vi "Pump Elapsed Time.vi"(11 "Pump Refs in":T1 {"Pump Info"."Direction" items=["CW", "CCW"]; "Pump Info"."Speed" format="%03.0f"}) -> (1 "Time has Elapsed":bool, 3 "Pump Refs in":T1 {"Pump Info"."Direction" items=["CW", "CCW"]; "Pump Info"."Speed" format="%03.0f"}, 4 "Elapsed Time (s)":dbl)   [LabVIEW 2020, in "Pump.lvlib"]
uses:
  Pump.lvlib
  Pump Hardware Configuration.ctl
  support/Message Queue/Message Cluster.ctl
  support/Message Queue/Message Queue.lvlib
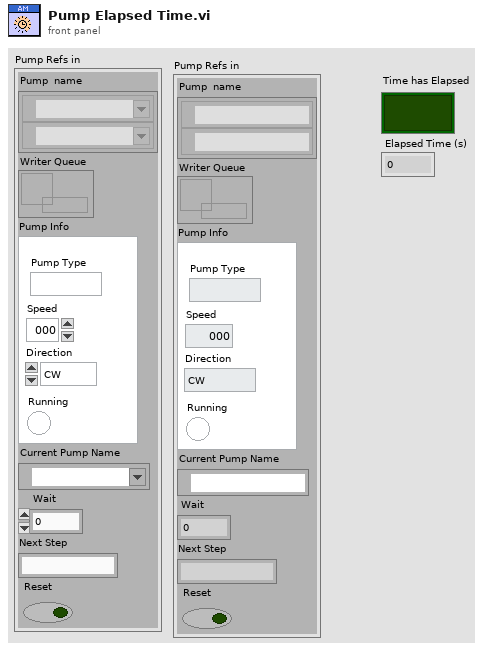
[diagram p1: front panel]
types:
  T1 = typedef "Pump.lvlib/Pump Hardware Configuration.ctl" = cluster{"Pump  name":refnum<visa-resource-name>[], "Writer Queue":refnum<queue>, "Pump Info":cluster{"Pump Type":string, "Speed":i32, "Direction":u16, "Running":bool}, "Current Pump Name":refnum<visa-resource-name>, "Wait":dbl, "Next Step":string, "Reset":bool}
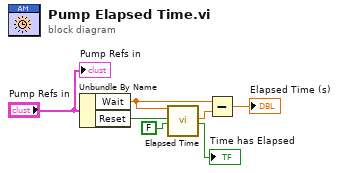
[diagram p0: block diagram]
diagram:
  n1 = Unbundle By Name("Pump Refs in") -> ("Wait"=w1:dbl, "Reset"=w5:bool)
  n2 = call "Elapsed Time"("Time Target (s)"=w1, "Reset"=w5, "Auto Reset"=FALSE) -> ("Elapsed Time (s)"=w3:dbl, "Time has Elapsed"=→"Time has Elapsed":bool)  [unwired: 9 in, 6 out]
  n3 = Subtract(x=w1, y=w3) -> (x-y=→"Elapsed Time (s)":dbl)
  "Pump Refs in" <- "Pump Refs in"
